vi "Stats Measurement Saver.vi"(0 "Dynamic Data":dynamicdata(waveform), 1 "OK Button":bool) -> ()   [LabVIEW 2023]
uses:
  <vilib>/express/express shared/transition.llb/Dynamic To Waveform Array.vi
  <vilib>/express/express signal manip/GetorSetDDTAttributes/Set DDT Attributes/SetT0.vi
  <vilib>/express/express shared/transition.llb/Waveform Array To Dynamic.vi
  <vilib>/express/express signal manip/GetorSetDDTAttributes/Set DDT Attributes/Set DDT Properties.xnode
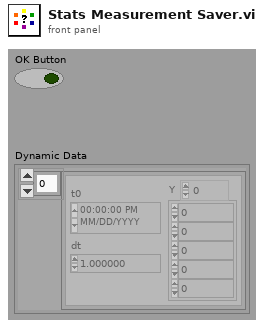
[diagram p1: front panel]
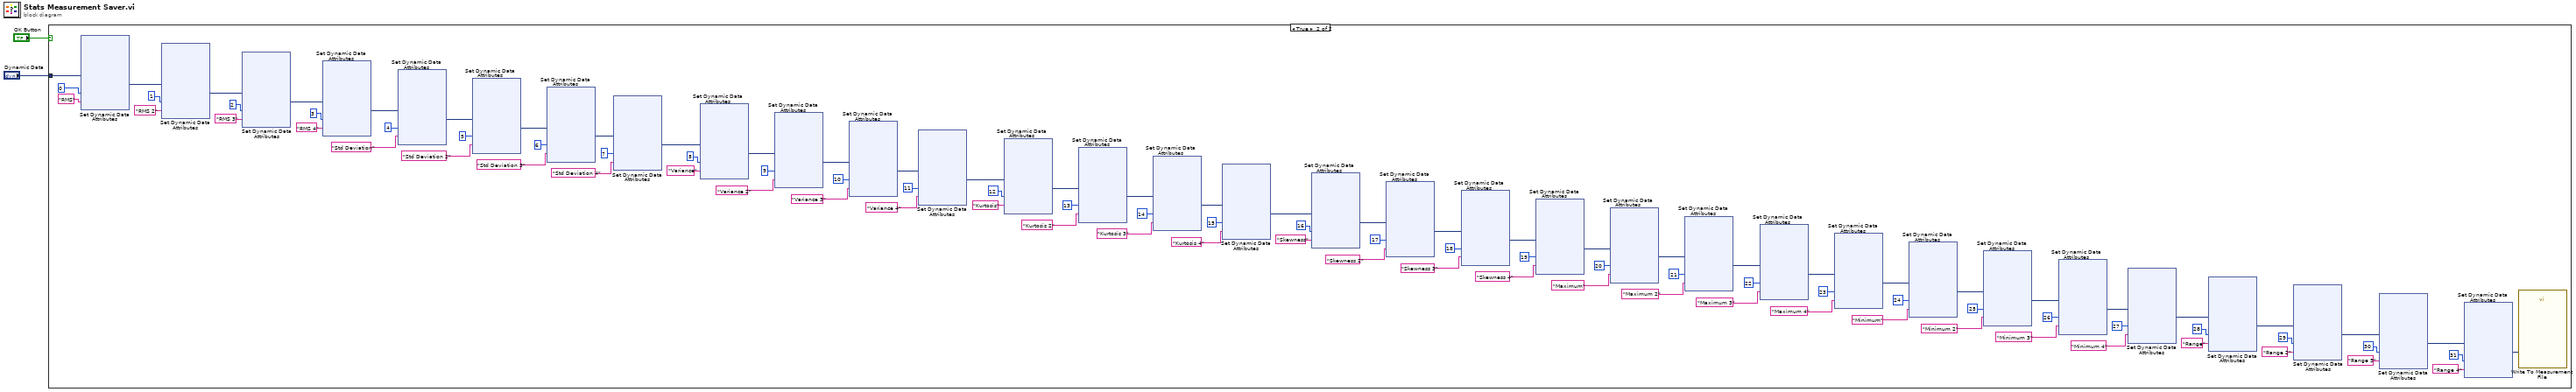
[diagram p0: block diagram]
diagram:
  n1 = case shown="True" "OK Button" {
    tunnel: "Dynamic Data" -> [_ w99]
    frame False {
    }
    frame True {
      n2 = xnode "Set Dynamic Data Attributes"("Signals In"=w99, "Signal Index"=0, "Signal Name"="RMS") -> ("Signals Out"=w96:dynamicdata)  [unwired: 1 in, 1 out]
      n3 = xnode "Set Dynamic Data Attributes"("Signals In"=w96, "Signal Index"=1, "Signal Name"="RMS 2") -> ("Signals Out"=w91:dynamicdata)  [unwired: 1 in, 1 out]
      n4 = xnode "Set Dynamic Data Attributes"("Signals In"=w91, "Signal Index"=2, "Signal Name"="RMS 3") -> ("Signals Out"=w90:dynamicdata)  [unwired: 1 in, 1 out]
      n5 = xnode "Set Dynamic Data Attributes"("Signals In"=w90, "Signal Index"=3, "Signal Name"="RMS 4") -> ("Signals Out"=w85:dynamicdata)  [unwired: 1 in, 1 out]
      n6 = xnode "Set Dynamic Data Attributes"("Signals In"=w85, "Signal Index"=4, "Signal Name"="Std Deviation") -> ("Signals Out"=w84:dynamicdata)  [unwired: 1 in, 1 out]
      n7 = xnode "Set Dynamic Data Attributes"("Signals In"=w84, "Signal Index"=5, "Signal Name"="Std Deviation 2") -> ("Signals Out"=w79:dynamicdata)  [unwired: 1 in, 1 out]
      n8 = xnode "Set Dynamic Data Attributes"("Signals In"=w79, "Signal Index"=6, "Signal Name"="Std Deviation 3") -> ("Signals Out"=w78:dynamicdata)  [unwired: 1 in, 1 out]
      n9 = xnode "Set Dynamic Data Attributes"("Signals In"=w78, "Signal Index"=7, "Signal Name"="Std Deviation 4") -> ("Signals Out"=w75:dynamicdata)  [unwired: 1 in, 1 out]
      n10 = xnode "Set Dynamic Data Attributes"("Signals In"=w75, "Signal Index"=8, "Signal Name"="Variance") -> ("Signals Out"=w72:dynamicdata)  [unwired: 1 in, 1 out]
      n11 = xnode "Set Dynamic Data Attributes"("Signals In"=w72, "Signal Index"=9, "Signal Name"="Variance 2") -> ("Signals Out"=w69:dynamicdata)  [unwired: 1 in, 1 out]
      n12 = xnode "Set Dynamic Data Attributes"("Signals In"=w69, "Signal Index"=10, "Signal Name"="Variance 3") -> ("Signals Out"=w66:dynamicdata)  [unwired: 1 in, 1 out]
      n13 = xnode "Set Dynamic Data Attributes"("Signals In"=w66, "Signal Index"=11, "Signal Name"="Variance 4") -> ("Signals Out"=w63:dynamicdata)  [unwired: 1 in, 1 out]
      n14 = xnode "Set Dynamic Data Attributes"("Signals In"=w63, "Signal Index"=12, "Signal Name"="Kurtosis") -> ("Signals Out"=w56:dynamicdata)  [unwired: 1 in, 1 out]
      n15 = xnode "Set Dynamic Data Attributes"("Signals In"=w56, "Signal Index"=13, "Signal Name"="Kurtosis 2") -> ("Signals Out"=w55:dynamicdata)  [unwired: 1 in, 1 out]
      n16 = xnode "Set Dynamic Data Attributes"("Signals In"=w55, "Signal Index"=14, "Signal Name"="Kurtosis 3") -> ("Signals Out"=w54:dynamicdata)  [unwired: 1 in, 1 out]
      n17 = xnode "Set Dynamic Data Attributes"("Signals In"=w54, "Signal Index"=15, "Signal Name"="Kurtosis 4") -> ("Signals Out"=w51:dynamicdata)  [unwired: 1 in, 1 out]
      n18 = xnode "Set Dynamic Data Attributes"("Signals In"=w51, "Signal Index"=16, "Signal Name"="Skewness") -> ("Signals Out"=w48:dynamicdata)  [unwired: 1 in, 1 out]
      n19 = xnode "Set Dynamic Data Attributes"("Signals In"=w48, "Signal Index"=17, "Signal Name"="Skewness 2") -> ("Signals Out"=w45:dynamicdata)  [unwired: 1 in, 1 out]
      n20 = xnode "Set Dynamic Data Attributes"("Signals In"=w45, "Signal Index"=18, "Signal Name"="Skewness 3") -> ("Signals Out"=w42:dynamicdata)  [unwired: 1 in, 1 out]
      n21 = xnode "Set Dynamic Data Attributes"("Signals In"=w42, "Signal Index"=19, "Signal Name"="Skewness 4") -> ("Signals Out"=w4:dynamicdata)  [unwired: 1 in, 1 out]
      n22 = xnode "Set Dynamic Data Attributes"("Signals In"=w4, "Signal Index"=20, "Signal Name"="Maximum") -> ("Signals Out"=w37:dynamicdata)  [unwired: 1 in, 1 out]
      n23 = xnode "Set Dynamic Data Attributes"("Signals In"=w37, "Signal Index"=21, "Signal Name"="Maximum 2") -> ("Signals Out"=w34:dynamicdata)  [unwired: 1 in, 1 out]
      n24 = xnode "Set Dynamic Data Attributes"("Signals In"=w34, "Signal Index"=22, "Signal Name"="Maximum 3") -> ("Signals Out"=w31:dynamicdata)  [unwired: 1 in, 1 out]
      n25 = xnode "Set Dynamic Data Attributes"("Signals In"=w31, "Signal Index"=23, "Signal Name"="Maximum 4") -> ("Signals Out"=w28:dynamicdata)  [unwired: 1 in, 1 out]
      n26 = xnode "Set Dynamic Data Attributes"("Signals In"=w28, "Signal Index"=24, "Signal Name"="Minimum") -> ("Signals Out"=w25:dynamicdata)  [unwired: 1 in, 1 out]
      n27 = xnode "Set Dynamic Data Attributes"("Signals In"=w25, "Signal Index"=25, "Signal Name"="Minimum 2") -> ("Signals Out"=w20:dynamicdata)  [unwired: 1 in, 1 out]
      n28 = xnode "Set Dynamic Data Attributes"("Signals In"=w20, "Signal Index"=26, "Signal Name"="Minimum 3") -> ("Signals Out"=w19:dynamicdata)  [unwired: 1 in, 1 out]
      n29 = xnode "Set Dynamic Data Attributes"("Signals In"=w19, "Signal Index"=27, "Signal Name"="Minimum 4") -> ("Signals Out"=w16:dynamicdata)  [unwired: 1 in, 1 out]
      n30 = xnode "Set Dynamic Data Attributes"("Signals In"=w16, "Signal Index"=28, "Signal Name"="Range") -> ("Signals Out"=w13:dynamicdata)  [unwired: 1 in, 1 out]
      n31 = xnode "Set Dynamic Data Attributes"("Signals In"=w13, "Signal Index"=29, "Signal Name"="Range 2") -> ("Signals Out"=w10:dynamicdata)  [unwired: 1 in, 1 out]
      n32 = xnode "Set Dynamic Data Attributes"("Signals In"=w10, "Signal Index"=30, "Signal Name"="Range 3") -> ("Signals Out"=w7:dynamicdata)  [unwired: 1 in, 1 out]
      n33 = xnode "Set Dynamic Data Attributes"("Signals In"=w7, "Signal Index"=31, "Signal Name"="Range 4") -> ("Signals Out"=w3:dynamicdata)  [unwired: 1 in, 1 out]
      n34 = call "Write To Measurement File"("Signals"=w3) -> ()  [unwired: 16 in, 3 out]
    }
  }
